vi "Modtag_string.vi"() -> ()   [LabVIEW 2018]
uses:
  <vilib>/myRIO/Instrument Drivers/Onboard IO/UART/typedef/VISA Configuration.ctl
  <vilib>/Instr/_visa.llb/VISA Configure Serial Port (Instr).vi
  <vilib>/myRIO/Instrument Drivers/Onboard IO/UART/UART.lvlib
panel:
  in  "stop":bool
  out "array":u8[](array[numeric])
  out "error out":errorcluster
  in  "error in (no error)":errorcluster
  out "Characters Read":string
  in  "Character Count":u32
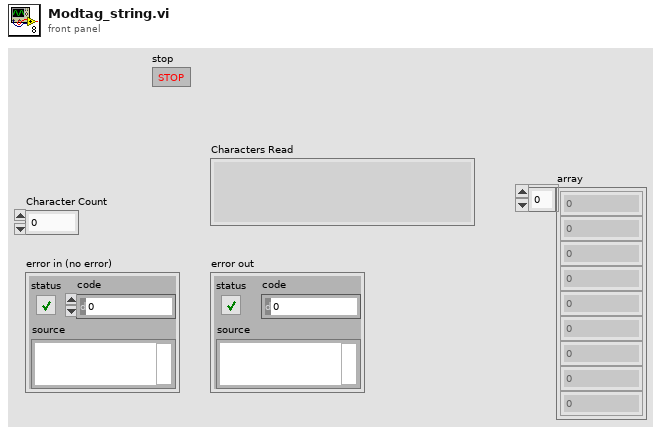
[diagram p1: front panel]
types:
  T1 = typedef "UART.lvlib/VISA Configuration.ctl" = cluster{"baud rate (9600)":u32, "data bits (8)":u16, "parity (0:none)":enum16{"None", "Odd", "Even", "Mark", "Space"}, "stop bits (10: 1 bit)":u16, "flow control (0:none)":u16, "termination char\n(0xA = '\\n' = LF) ":u8, "Enable Termination\nChar (T)":bool, "timeout (10sec)":u32}
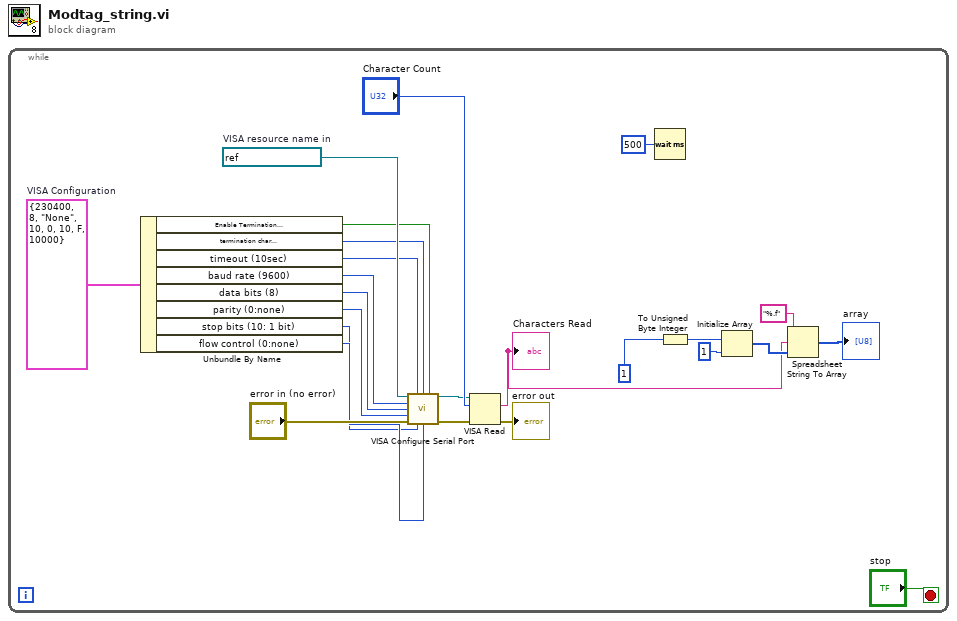
[diagram p0: block diagram]
diagram:
  n1 = while {
    stop <- "stop" stop-if-true
    w23 = T1 {"baud rate (9600)"=230400, "data bits (8)"=8, "parity (0:none)"=enum."None", "stop bits (10: 1 bit)"=10, "flow control (0:none)"=0, "termination char\n(0xA = '\\n' = LF) "=10, "Enable Termination\nChar (T)"=FALSE, "timeout (10sec)"=10000}  # VISA Configuration
    w24 = refnum<visa-resource-name> "ASRL1::INSTR"  # VISA resource name in
    n2 = Unbundle By Name(w23) -> ("Enable Termination\nChar (T)"=w17:bool, "termination char\n(0xA = '\\n' = LF)"=w16:u8, "timeout (10sec)"=w15:u32, "baud rate (9600)"=w10:u32, "data bits (8)"=w11:u16, "parity (0:none)"=w12:enum16{"None", "Odd", "Even", "Mark", "Space"}, "stop bits (10: 1 bit)"=w13:u16, "flow control (0:none)"=w14:u16)
    n3 = call-poly "VISA Configure Serial Port"("VISA resource name"=w24, "timeout (10sec)"=w15, "termination char\n(0xA = '\\n' = LF)"=w16, "Enable Termination\nChar (T)"=w17, "baud rate (9600)"=w10, "data bits (8)"=w11, "parity (0:none)"=w12, "error in (no error)"="error in (no error)", "stop bits (10: 1 bit)"=w13, "flow control (0:none)"=w14) -> ("VISA resource name out"=w20:refnum<visa-resource-name>, "error out"=w19:errorcluster)  [unwired: 4 in]
    n4 = VISA Read(VISA resource name=w20, byte count="Character Count", error in (no error)=w19) -> (read buffer=w4:string, error out=→"error out":errorcluster)  [unwired: 2 out]
    "Characters Read" <- w4
    n5 = Wait (ms)(milliseconds to wait=u32 500) -> ()  [unwired: 1 out]
    n6 = To Unsigned Byte Integer(number=u8 1) -> (unsigned 8bit integer=w7:u8)
    n7 = Initialize Array(w7, 1 ("dimension size")) -> (w5:u8[])
    n8 = Spreadsheet String To Array(format string="%.f", spreadsheet string=w4, array type (2D Dbl)=w5) -> (array=→"array":u8[])  [unwired: 1 in]
  }
